vi "数据处理2.vi"(6 "原始数据文件名":string, 7 "去噪信号保存的文件名":string, 8 "sym":string, 9 "数组中的数据（输入）":dbl[](array[numeric]), 11 "lev":i32) -> (1 "字符串（输出）":string, 2 "特征值（输出）":dbl[][](array[numeric]), 3 "去噪后波形图":dbl[][](graph))   [LabVIEW 2018]
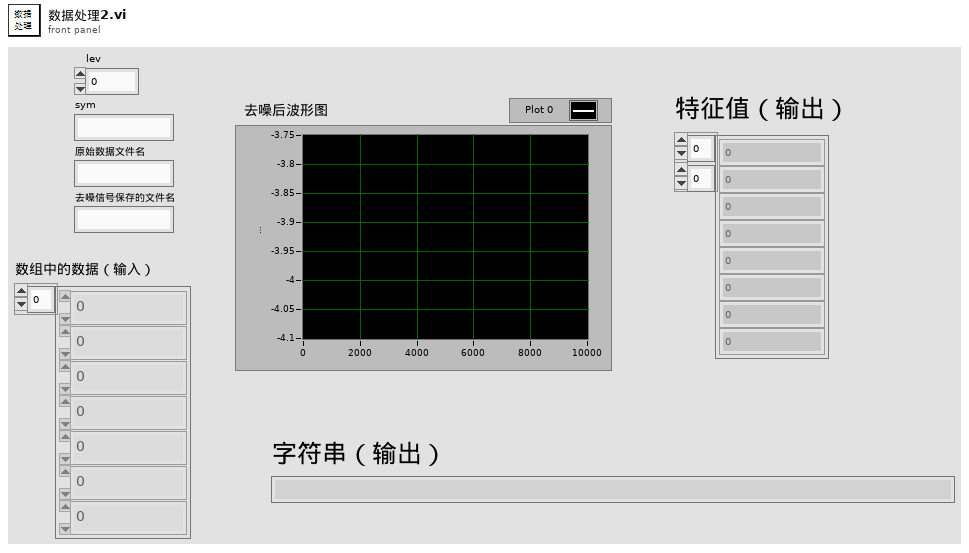
[diagram p1: front panel]
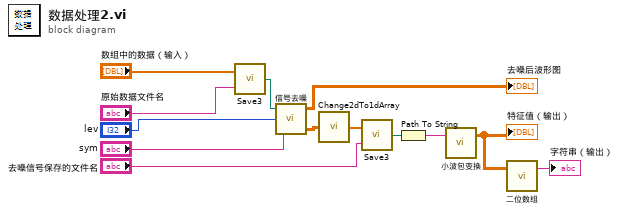
[diagram p0: block diagram]
diagram:
  n1 = call "Save3.vi"("要保存的文件名（输入）"="原始数据文件名", "数组中的数据（输入）"="数组中的数据（输入）") -> ("文件保存路径（输出）"=w12:path)
  n2 = call "信号去噪.vi"("字符串"="sym", "数值"="lev", "文件路径（输入）"=w12) -> ("去噪后数据输出"=w8:dbl[][], "去噪后波形图（输出）"=→"去噪后波形图":dbl[][])  [unwired: 1 in]
  n3 = call "Change2dTo1dArray.vi"("AI2去噪后数据"=w8) -> ("AI2一维数组"=w7:dbl[])
  n4 = call "Save3.vi"("要保存的文件名（输入）"="去噪信号保存的文件名", "数组中的数据（输入）"=w7) -> ("文件保存路径（输出）"=w10:path)
  n5 = Path To String(path=w10) -> (string=w9:string)
  n6 = call "小波包变换.vi"("数据文件路径（输入）"=w9) -> ("特征值（输出）"=w5:dbl[][])  [unwired: 2 in]
  "特征值（输出）" <- w5
  n7 = call "二位数组.vi"("二位数组（输入）"=w5) -> ("字符串（输出）"=→"字符串（输出）":string)  [unwired: 1 in, 1 out]
